vi "Matrix_Block.vi"(6 "StartColumn":i32, 8 "StartRow":i32, 9 "Columns":i32, 10 "Rows":i32, 11 "input matrix":T1) -> (3 "output matrix":T1)   [LabVIEW 2019, in "Trajectory_Library.lvlib"]
doc: "Extracts a matrix of a given size and start position with new underlying storage.\n \nInputs:\n - input matrix -- The input matrix\n - Rows -- Number of rows to extract.\n - Columns -- Number of columns to extract.\n - startingRow -- The starting row of the extracted matrix.\n - startingCol -- The starting column of the extracted matrix.\n\nOutputs:\n - output matrix -- The extracted matrix."
uses:
  Trajectory_Library.lvlib
  <vilib>/Analysis/Matrix/Datatypes/RealMatrix.ctl
  MatBuilder_Create.vi
  <vilib>/Analysis/Matrix/NI_Matrix.lvlib
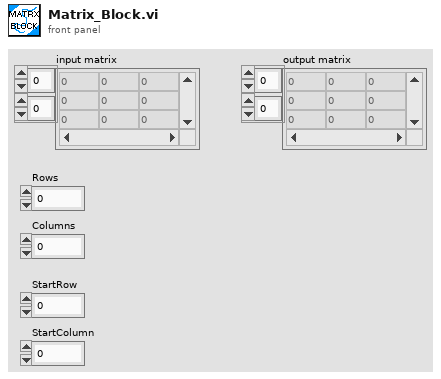
[diagram p1: front panel]
types:
  T1 = typedef "NI_Matrix.lvlib/RealMatrix.ctl" = dbl[][]
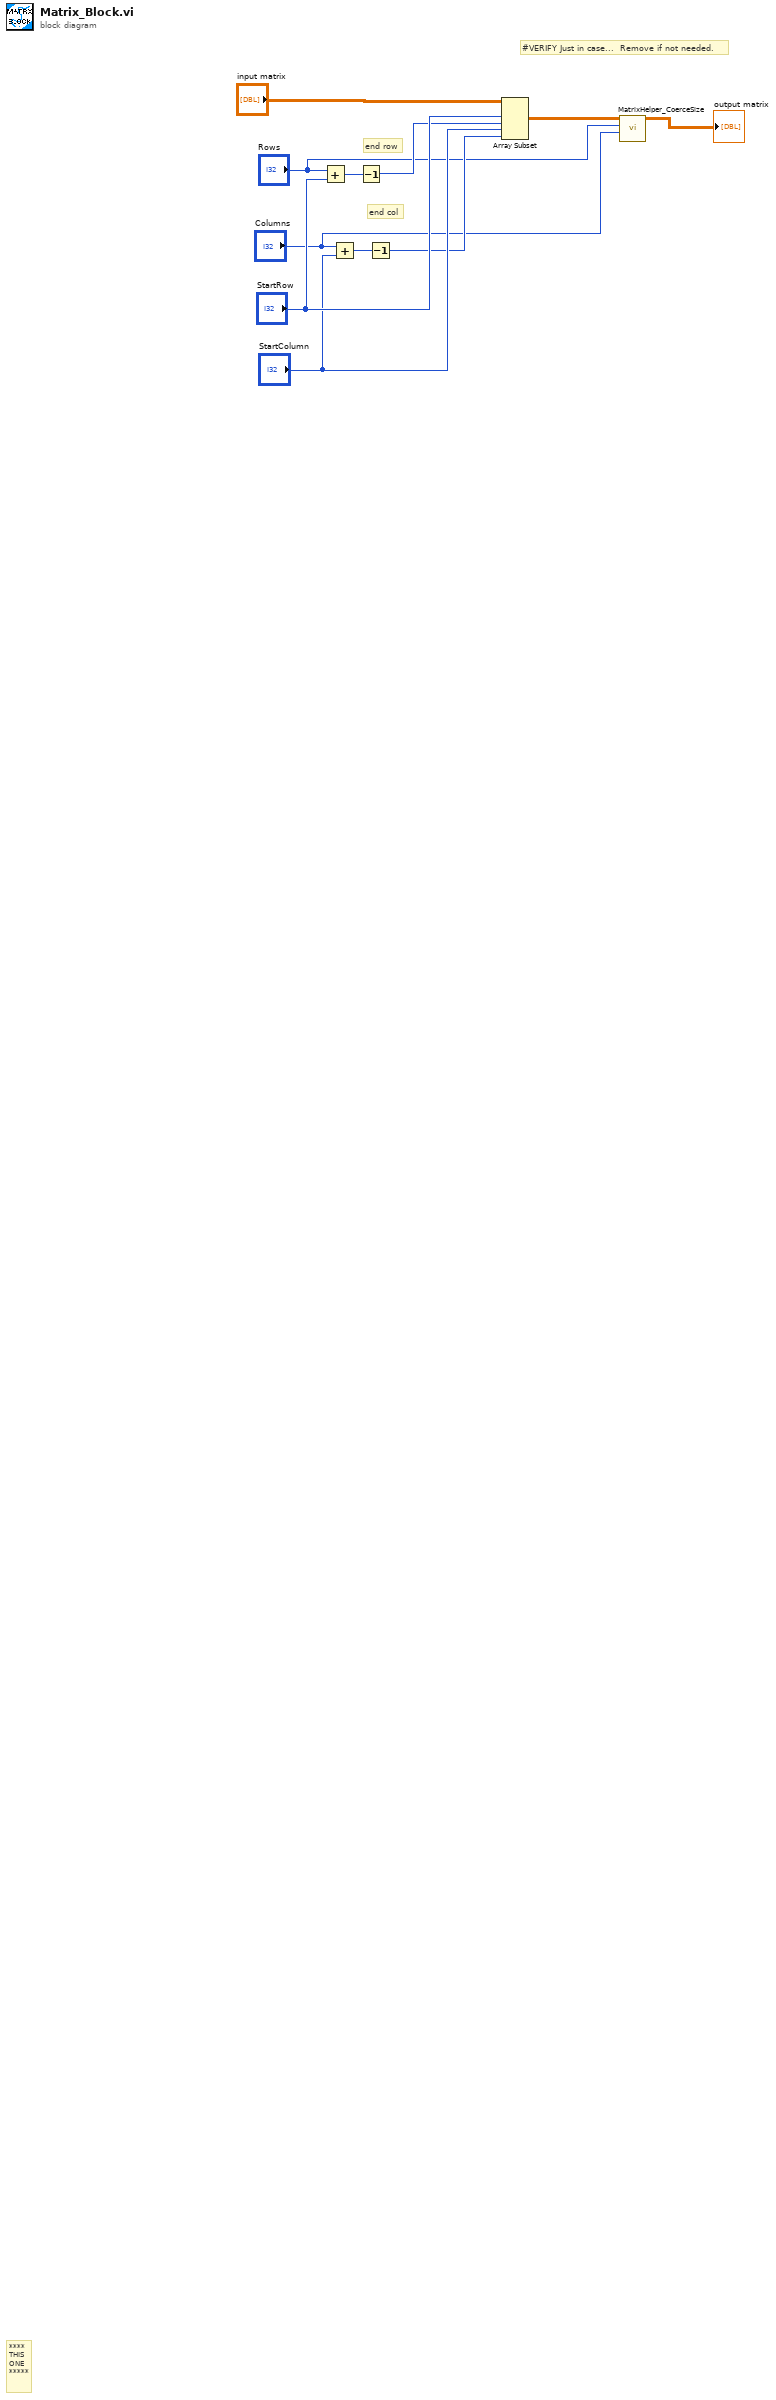
[diagram p0: block diagram]
diagram:
  # "#VERIFY Just in case...  Remove if not needed."
  # "end col"
  # "end row"
  # "****\nTHIS\nONE\n*****"
  n1 = Add(x="Rows", y="StartRow") -> (x+y=w8:i32)
  n2 = Add(x="Columns", y="StartColumn") -> (x+y=w7:i32)
  n3 = Decrement(x=w8) -> (x-1=w5:i32)
  n4 = Decrement(x=w7) -> (x-1=w4:i32)
  n5 = Array Subset(array="input matrix", index (row)="StartRow", length (row)=w5, index (col)="StartColumn", length (col)=w4) -> (w3:T1)
  n6 = call "MatrixHelper_CoerceSize.vi"("Columns"="Columns", "Rows"="Rows", "input matrix"=w3) -> ("output matrix"=→"output matrix":T1)  [unwired: 7 in, 1 out]
